vi "纳清浊度电极校准.vi"() -> ()   [LabVIEW 2016, in "斯坦道多参数.lvlib"]
uses:
  <vilib>/Utility/miscctls.llb/LVPointTypeDef.ctl
  <vilib>/Utility/miscctls.llb/LVPositionTypeDef.ctl
  <vilib>/Analysis/NI_AALBase.lvlib
panel:
  out "清扫间隔":u16
  out "清扫次数":u16
  in  "清扫模式":u16(ring) items=["自动清扫", "手动清扫", "启动一次清扫"]
  out "滤波设定":sgl
  out "第三点信号值":dbl
  out "第二点信号值":dbl
  out "第一点信号值":dbl
  in  "量程":u16(ring) items=["0-100", "0-500", "0-2000", "0-4000"]
  out "报警信息":string
  out "通讯状态":string
  out "第三点校准值":dbl
  out "标液3":sgl
  out "第二点校准值":dbl
  out "第一点校准值":dbl
  in  "校准停止":bool
  in  "校准启动":bool
  in  "校准模式":u16(ring)=1 items=["两点校准", "单点校准", "三点校准"]
  out "最小值":sgl format="%#.2f"
  out "最大值":sgl format="%#.2f"
  out "波形图表":dbl(graph) caption="历史曲线"
  out "mean":dbl caption="均值" format="%#.2f"
  out "standard deviation":dbl caption="标准差" format="%#.2f"
  out "变异系数":dbl format="%#.6f"
  out "测量值":sgl format="%#.2f"
  out "提示":string
  out "标液2":sgl
  out "标液1":sgl
  out "原始光强数值":u16 caption="信号值"
  out "温度":dbl format="%#.2f"
  # "浊度电极设定"
  # "℃"
  # "NTU"
  # "NTU"
  # "请选择校准模式:"
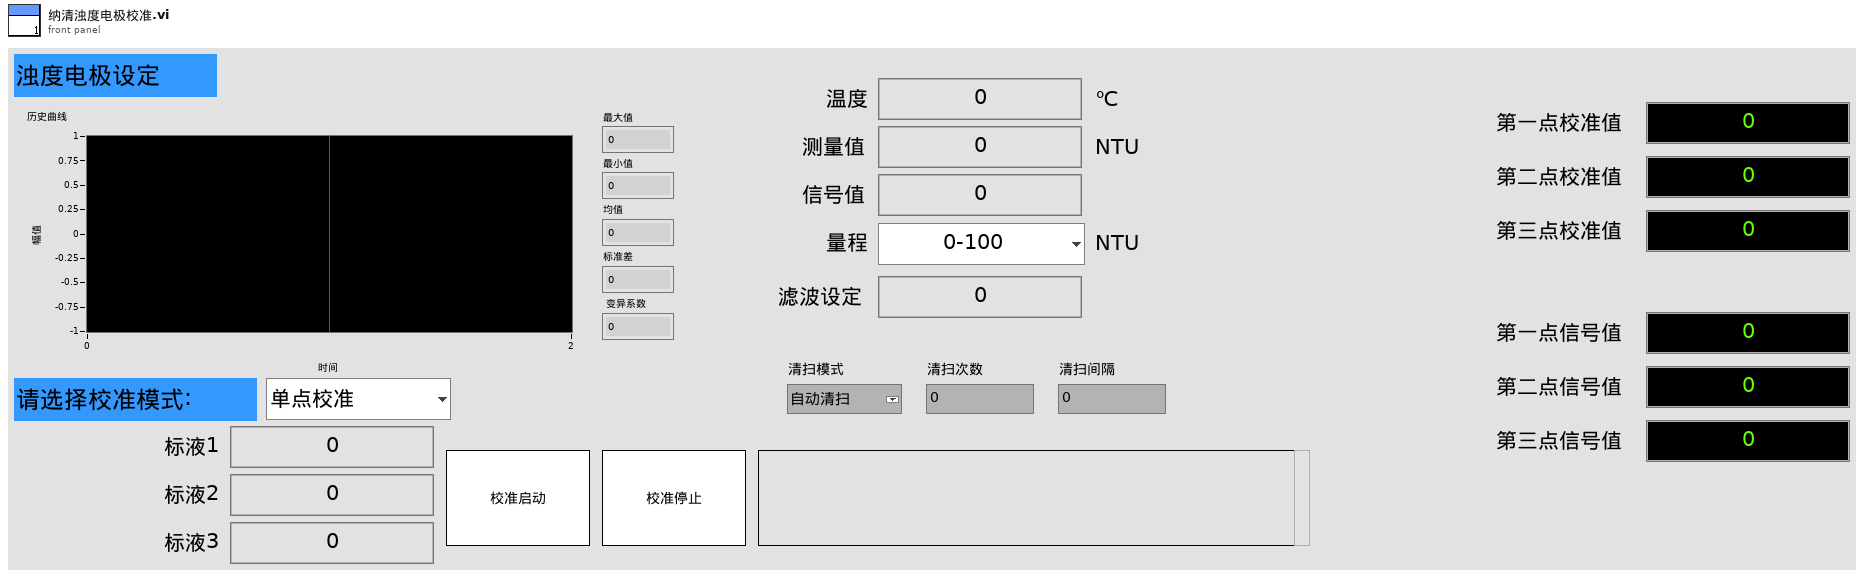
[diagram p1: front panel]
types:
  T1 = enum16{"pH", "DO", "Cond", "Turb", "ORP", "叶绿素a", "藻密度"}
  T2 = typedef "LVPointTypeDef.ctl" = cluster{"Horizontal":i16, "Vertical":i16}
  T3 = cluster{"报警码":u16, "浊度数值 NTU":sgl, "温度数据":sgl, "原始光强数值":u16, "量程":u16, "平均次数":u16, "清扫模式":u16, "清扫次数":u16, "清扫间隔分钟":u16, "0X000B_NC":string, "产品名称":string, "序列号":string, "硬件版本":string, "软件版本":string, "通讯地址":u16, "波特率":u16, "设备类型":u16, "0X0026_NC":string, "校准量程":u16, "第一点原始光强":u16, "第一点校准数据":sgl, "第二点原始光强":u16, "第二点校准数据":sgl, "第三点原始光强":u16, "第三点校准数据":sgl, "探头校准命令":u16, "温度校准参数":sgl, "温度校准命令":u16}
  T4 = cluster{"pH":u32, "DO":u32, "Cond":u32, "Turb":u32, "叶绿素a":u32, "藻密度":u32, "ORP":u32, "COD":u32}
  T5 = typedef "LVPositionTypeDef.ctl" = cluster{"Left":i32, "Top":i32}
  T6 = enum8{"Enabled", "Disabled", "Disabled and Grayed Out"}
  T7 = cluster{"ph":bool, "DO":bool, "Cond":bool, "Turb":bool, "叶绿素a":bool, "藻密度":bool, "ORP":bool, "COD":bool}
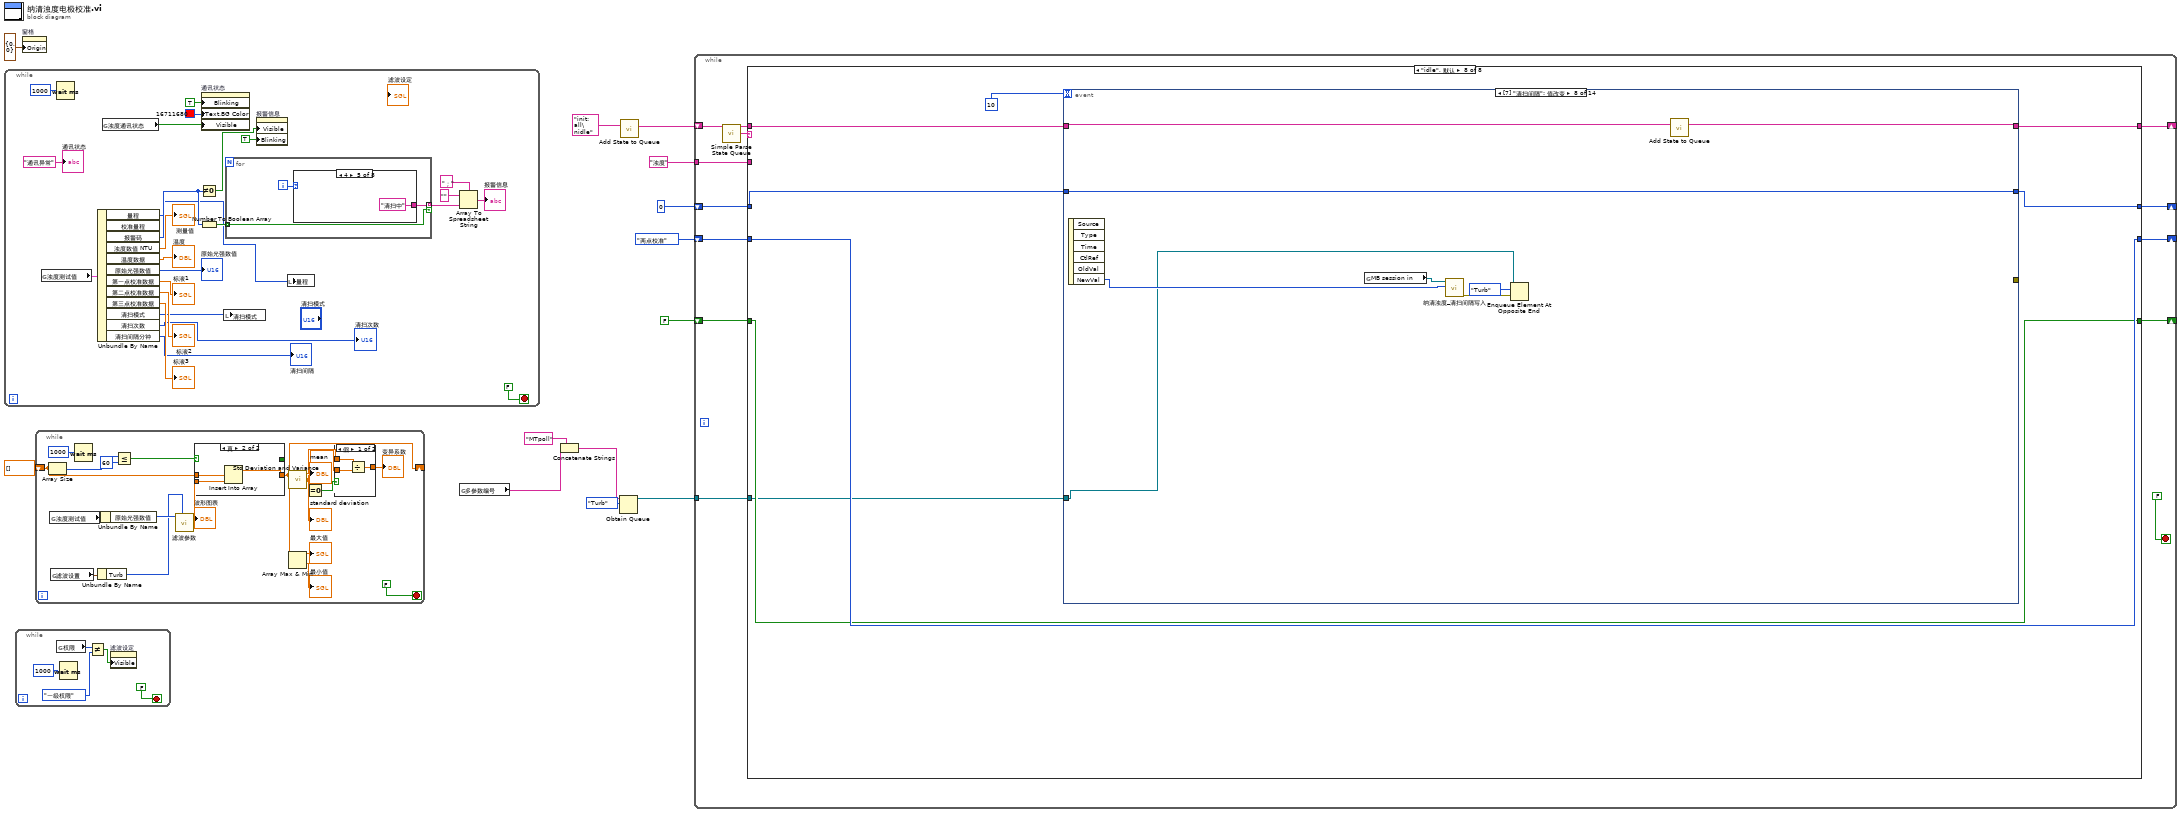
[diagram p0: block diagram]
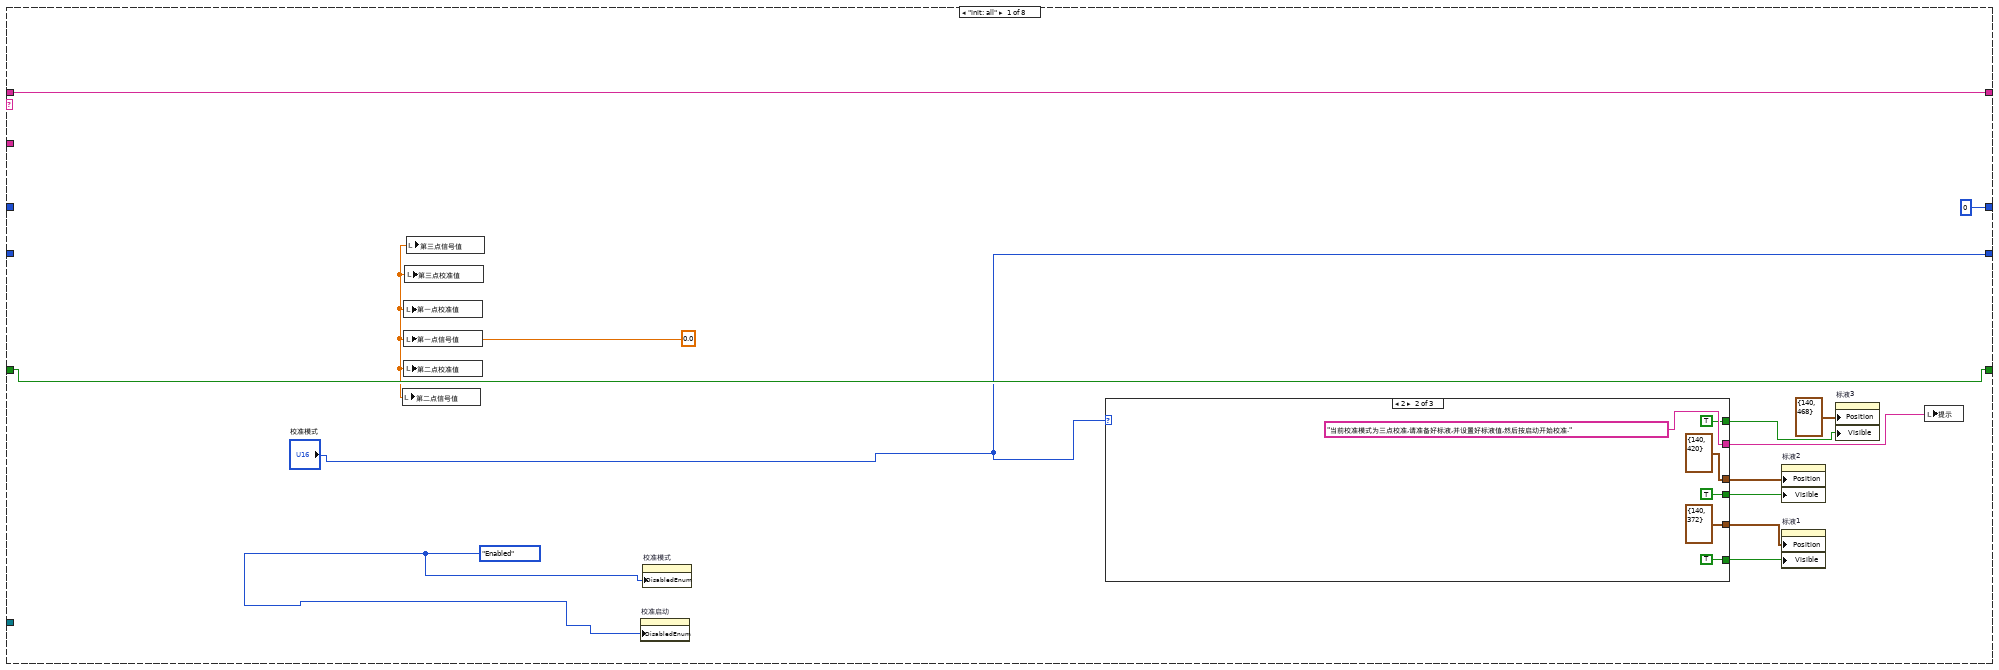
[diagram p2: hidden frame]
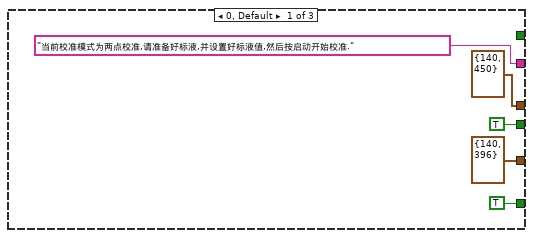
[diagram p3: hidden frame]
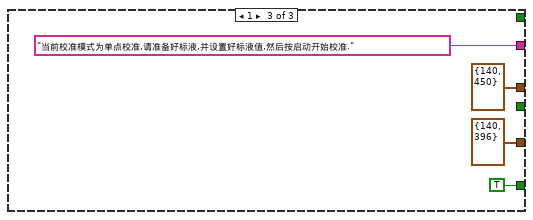
[diagram p4: hidden frame]
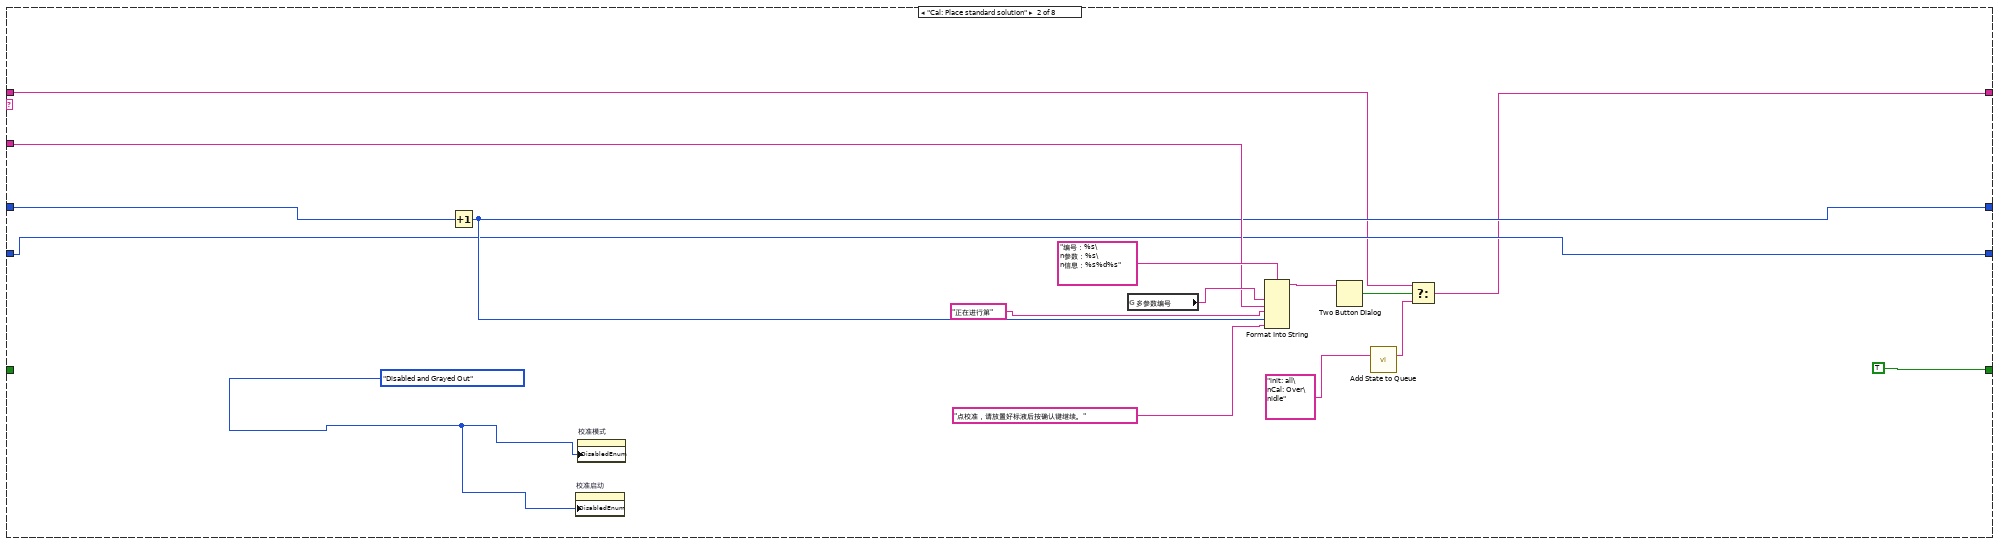
[diagram p5: hidden frame]
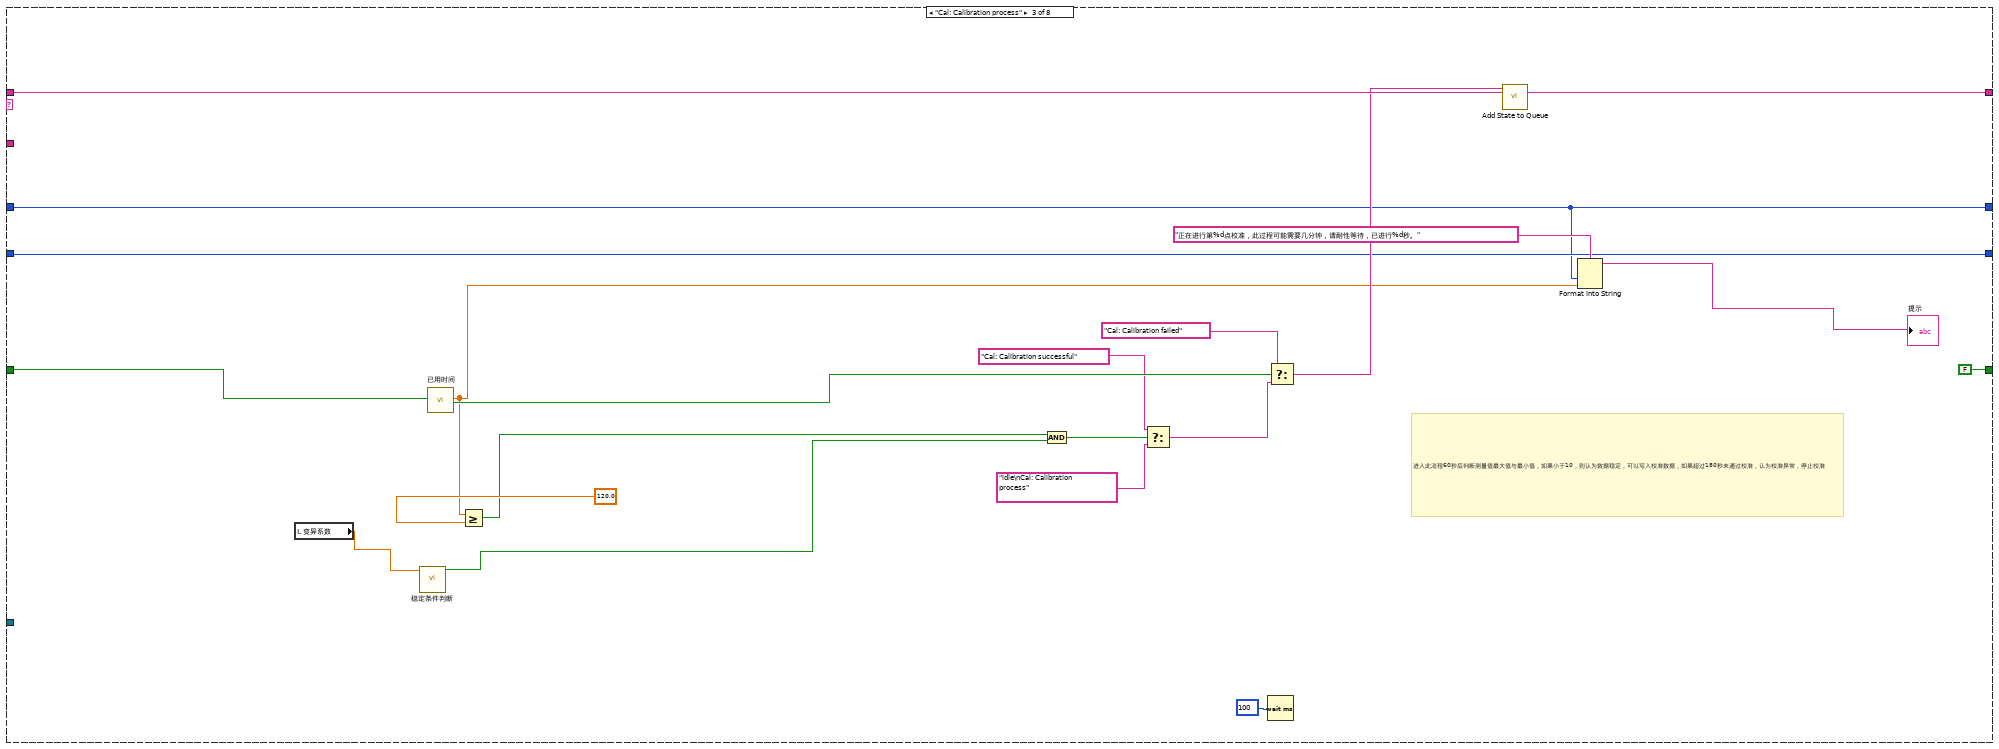
[diagram p6: hidden frame]
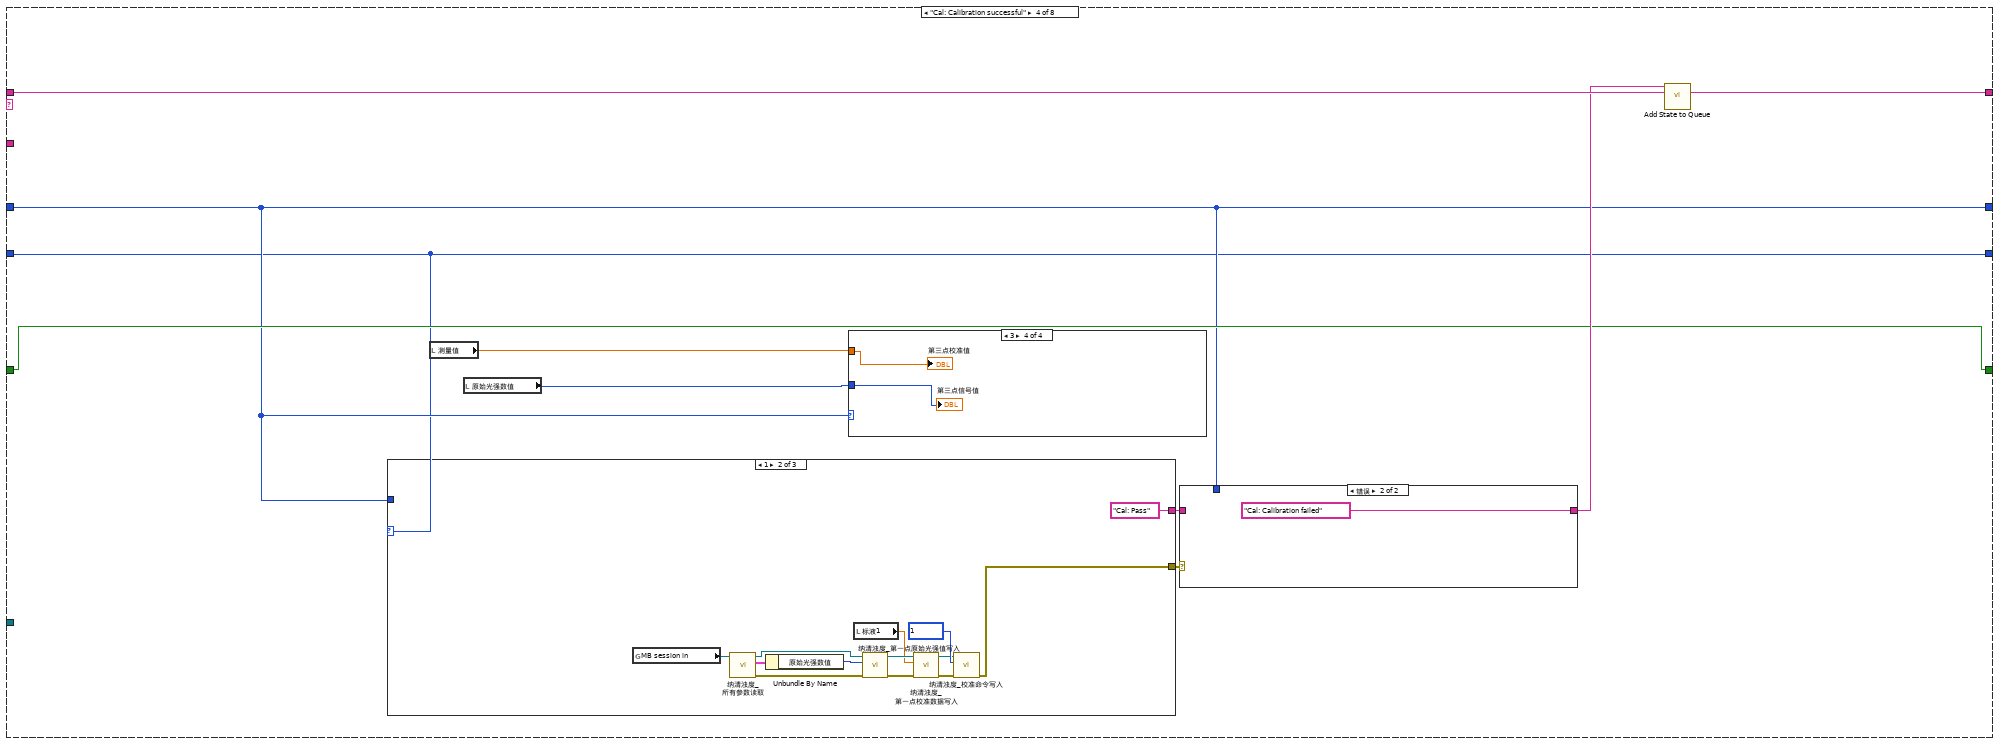
[diagram p7: hidden frame]
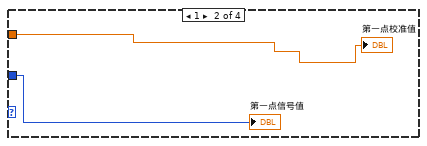
[diagram p9: hidden frame]
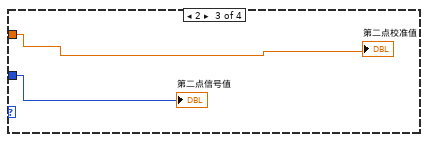
[diagram p10: hidden frame]
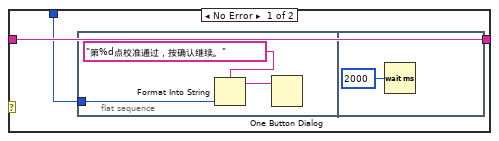
[diagram p11: hidden frame]
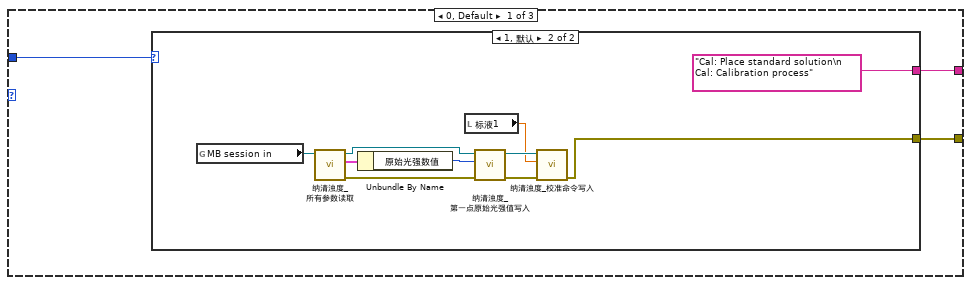
[diagram p12: hidden frame]
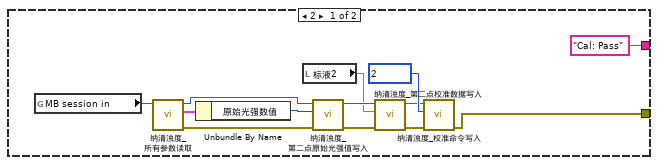
[diagram p13: hidden frame]
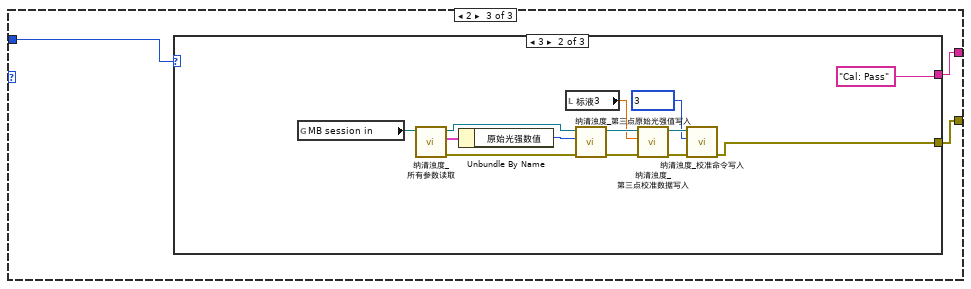
[diagram p14: hidden frame]
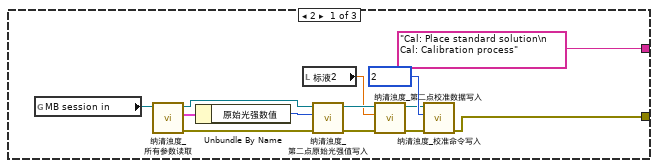
[diagram p15: hidden frame]
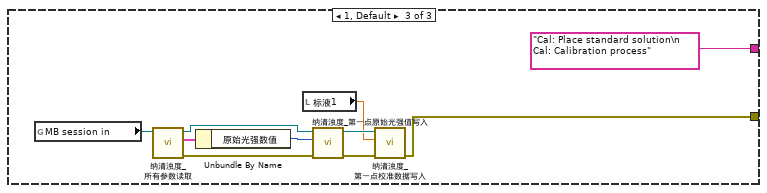
[diagram p16: hidden frame]
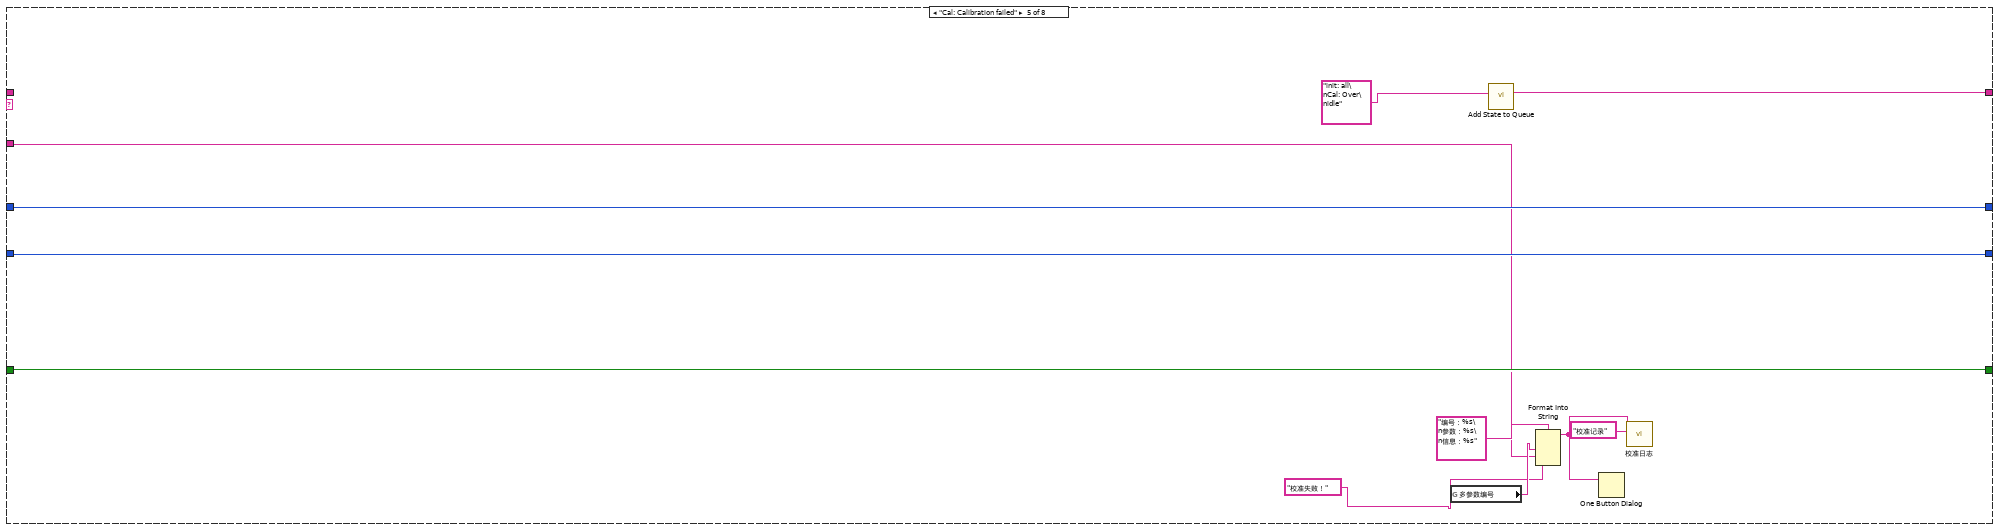
[diagram p17: hidden frame]
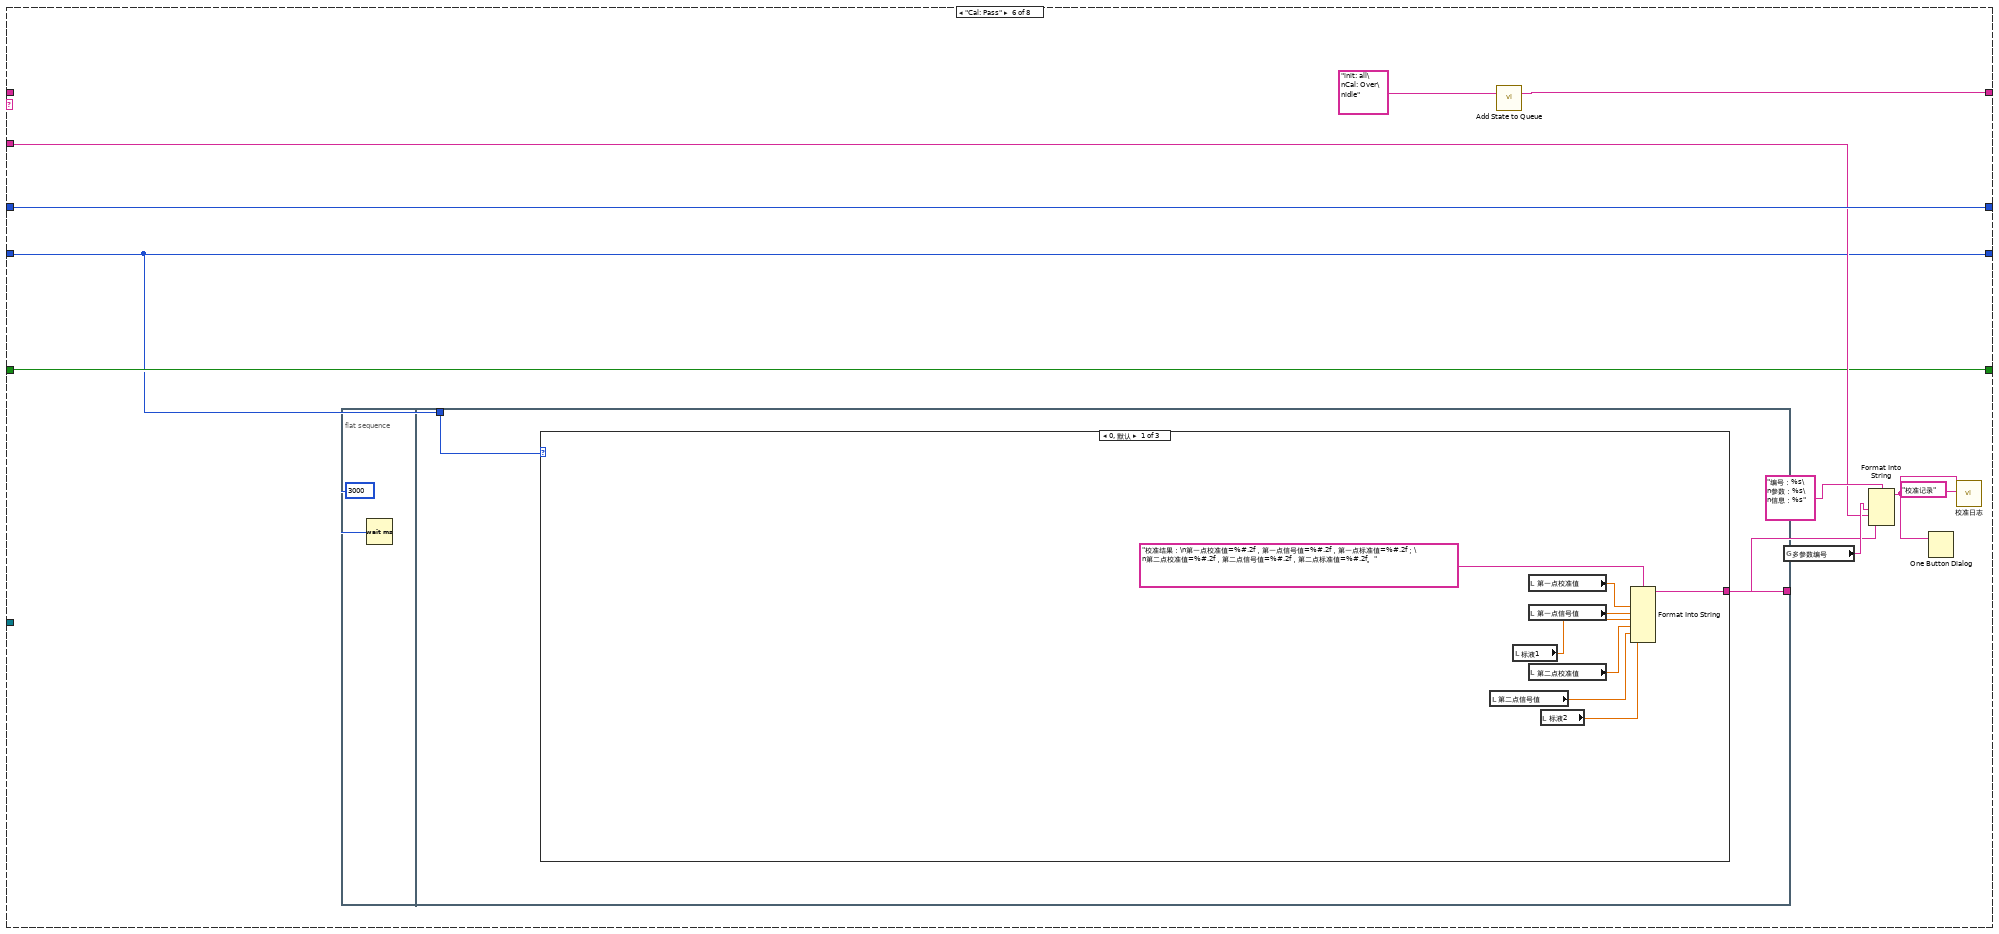
[diagram p18: hidden frame]
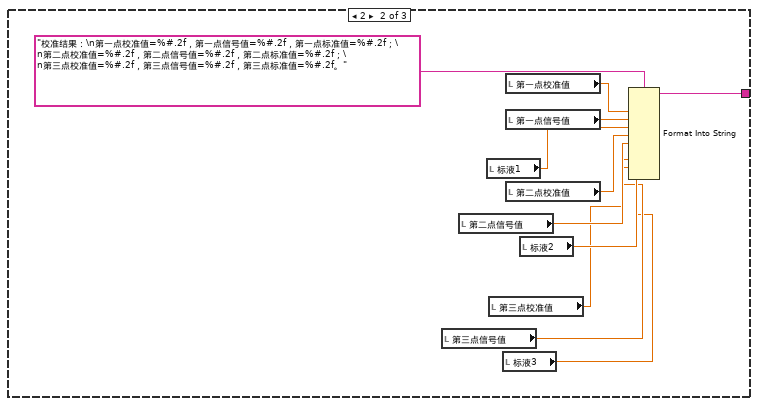
[diagram p19: hidden frame]
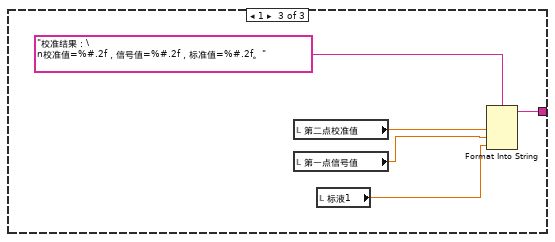
[diagram p20: hidden frame]
diagram:
  n1 = while {
    stop <- FALSE stop-if-true
    n2 = global read "纳清过程全局变量.vi" "浊度测试值"() -> (w36:T3)
    n3 = Wait (ms)(milliseconds to wait=u32 1000 ("等待时间（毫秒）")) -> ()  [unwired: 1 out]
    n4 = Unbundle By Name(w36) -> ("量程"=w17:u16, "报警码"=w18:u16, "浊度数值 NTU"=→"测量值":sgl, "温度数据"=→"温度":sgl, "原始光强数值"=→"原始光强数值":u16, "第一点校准数据"=→"标液1":sgl, "第二点校准数据"=→"标液2":sgl, "第三点校准数据"=→"标液3":sgl, "清扫模式"=w14:u16, "清扫次数"=→"清扫次数":u16, "清扫间隔分钟"=→"清扫间隔":u16)  [unwired: 1 out]
    n5 = global read "多参数全局变量.vi" "浊度通讯状态"() -> (w26:bool)
    n6 = Not Equal To 0?(x=w18) -> (x != 0?=w20:bool)
    n7 = Number To Boolean Array(number=w18) -> (Boolean array=w25:bool[])
    n8 = property on="通讯状态" class="Str"("Blinking"=TRUE ("闪烁"), "Text.BG Color"=u32 16711680, "Visible"=w26) -> ()  [unwired: 2 in, 2 out]
    n9 = local write "清扫模式"(w14) -> ()
    n10 = for {
      tunnel: w25 -> [w39] mode=indexing
      tunnel: [w40] -> w24 mode=indexing if=w39
      i -> [w41]
      n11 = case shown="4" w41 {
        tunnel: [_ "浊度超量程" "温度超量程" "光强信号超范围" "清扫中" "温度传感器故障" "电极故障" "内部电压基准故障"] -> w40
        frame Default {
        }
        frame 0 {
        }
        frame 2 {
        }
        frame 3 {
        }
        frame 4 {
        }
        frame 8 {
        }
        frame 9 {
        }
        frame 10 {
        }
      }
    }
    n12 = property on="报警信息" class="Str"("Visible"=w20, "Blinking"=TRUE ("闪烁")) -> ()  [unwired: 2 in, 2 out]
    n13 = local write "量程"(w17) -> ()
    n14 = Array To Spreadsheet String(delimiter (Tab)="；" ("分隔符(Tab)"), array=w24, 3:"" ("格式字符串")) -> (spreadsheet string=→"报警信息":string)
    "通讯状态" <- "通讯异常" ("当前串口")
  }
  n15 = while {
    stop <- FALSE stop-if-true
    n16 = global read "多参数全局变量.vi" "权限"() -> (w52:enum16{"一级权限", "二级权限", "三级权限"})
    n17 = Wait (ms)(milliseconds to wait=u32 1000 ("等待时间（毫秒）")) -> ()  [unwired: 1 out]
    n18 = Not Equal?(x=w52, y=enum16{"一级权限", "二级权限", "三级权限"}."一级权限") -> (x != y?=w49:bool)
    n19 = property on="滤波设定" class="DigNum (严格)"("Visible"=w49) -> ()  [unwired: 2 in, 2 out]
  }
  n20 = property on="窗格" class="Pane"("Origin"=T2 {"Horizontal"=0, "Vertical"=0} ("原点")) -> ()  [unwired: 2 in, 2 out]
  n21 = while {
    shift-right: [w61] -> _
    shift-left: sgl[] [] -> [w67]
    stop <- FALSE stop-if-true
    n22 = Array Size(array=w67) -> (size(s)=w69:i32)
    n23 = global read "纳清过程全局变量.vi" "浊度测试值"() -> (w58:T3)
    n24 = global read "断电保存变量.vi" "滤波设置"() -> (w55:T4)
    n25 = Wait (ms)(milliseconds to wait=u32 1000 ("等待时间（毫秒）")) -> ()  [unwired: 1 out]
    n26 = Unbundle By Name(w55) -> ("Turb"=w54:u32)
    n27 = Unbundle By Name(w58) -> ("原始光强数值"=w57:u16)
    n28 = Less Or Equal?(x=w69, y=60) -> (x <= y?=w68:bool)
    n29 = call "滤波参数.vi"("滤波次数"=w54, "x"=w57) -> ("mode"=w56:dbl)  [unwired: 9 in]
    "波形图表" <- w56
    n30 = case shown="真" w68 {
      tunnel: w67 -> [w80 w83]
      tunnel: w56 -> [w78 w82]
      tunnel: [w76 w81] -> w61
      tunnel: [TRUE _] -> _
      frame False {
        n31 = Replace Array Subset(array=w80, new element=w78) -> (w79:sgl[])  [unwired: 1 in]
        n32 = Rotate 1D Array(1:w79, 2:-1 ("n")) -> (0:w76:sgl[])
      }
      frame True {
        n33 = Insert Into Array(array=w83, new element=w82) -> (w81:sgl[])  [unwired: 1 in]
      }
    }
    n34 = call <vilib>:"Std Deviation and Variance.vi"("X"=w61) -> ("mean"=w65:dbl, "standard deviation"=w64:dbl)  [unwired: 1 in, 1 out]
    "mean" <- w65
    "standard deviation" <- w64
    n35 = Array Max & Min(array=w61) -> (max value=→"最大值":sgl, min value=→"最小值":sgl)  [unwired: 2 out]
    n36 = Equal To 0?(x=w65) -> (x = 0?=w66:bool)
    n37 = case shown="假" w66 {
      tunnel: w64 -> [w74 _]
      tunnel: [w73 _] -> w63
      tunnel: w65 -> [w72 _]
      frame False {
        n38 = Divide(x=w74, y=w72) -> (x/y=w73:dbl)
      }
      frame True {
      }
    }
    "变异系数" <- w63
  }
  n39 = global read "多参数全局变量.vi" "多参数编号"() -> (w2:string)
  n40 = Concatenate Strings("MTpoll" ("名称（未命名）"), w2) -> (w4:string)
  n41 = Obtain Queue(name (unnamed)=w4, element data type=T1."Turb" ("枚举")) -> (queue out=w1:refnum<queue>)  [unwired: 3 in, 2 out]
  n42 = call "Add State to Queue.vi"("State(s) In (\"\")"="init: all\nidle" ("State(s) In (\"\")")) -> ("States Out"=w10:string)  [unwired: 14 in]
  n43 = while {
    shift-right: [w92] -> _
    shift-left: w10 -> [w96]
    shift-right: [w89] -> _
    shift-left: 0 -> [w91]
    tunnel: "浊度" ("State(s) In (\"\")") -> [w90]
    shift-right: [w87] -> _
    shift-left: enum16{"两点校准", "单点校准", "三点校准"}."两点校准" ("校准模式") -> [w88]
    shift-right: [w85] -> _
    shift-left: FALSE -> [w86]
    tunnel: w1 -> [w84]
    stop <- FALSE stop-if-true
    n44 = call "Simple Parse State Queue.vi"("State Queue"=w96) -> ("Remain States"=w93:string, "Next State"=w94:string)  [unwired: 13 in]
    n45 = case shown="\"idle\", 默认" w94 {
      tunnel: w93 -> [w109 w128 w160 w169 _ _ w318 w326]
      tunnel: [w109 w127 w159 w168 w270 w275 w318 w325] -> w92
      tunnel: w91 -> [_ w136 w145 w163 w273 w284 w317 w323]
      tunnel: w90 -> [_ w137 _ _ w264 w280 _ _]
      tunnel: [0 w134 w145 w163 w273 w284 w317 w324] -> w89
      tunnel: w88 -> [_ w133 w146 w162 w272 w276 w316 w322]
      tunnel: ["校准模式" w133 w146 w162 w272 w276 w316 w322] -> w87
      tunnel: w86 -> [w107 _ w148 w164 w271 w279 w315 w320]
      tunnel: [w107 TRUE FALSE w164 w271 w279 w315 w320] -> w85
      tunnel: w84 -> [_ _ _ _ _ _ _ w319]
      frame "init: all" {
        w105 = T6."Enabled" ("禁用")
        w106 = 0.0 ("第一点校准值")
        n46 = local write "第二点信号值"(w106) -> ()
        n47 = local write "第一点校准值"(w106) -> ()
        n48 = local write "第一点信号值"(w106) -> ()
        n49 = local write "第二点校准值"(w106) -> ()
        n50 = local write "第三点校准值"(w106) -> ()
        n51 = local write "第三点信号值"(w106) -> ()
        n52 = property on="校准启动" class="Bool"("DisabledEnum"=w105) -> ()  [unwired: 2 in, 2 out]
        n53 = property on="校准模式" class="Ring (严格)"("DisabledEnum"=w105) -> ()  [unwired: 2 in, 2 out]
        n54 = case shown="2" "校准模式" {
          tunnel: ["当前校准模式为两点校准,请准备好标液,并设置好标液值,然后按启动开始校准." ("提示") "当前校准模式为三点校准,请准备好标液,并设置好标液值,然后按启动开始校准." ("提示") "当前校准模式为单点校准,请准备好标液,并设置好标液值,然后按启动开始校准." ("提示")] -> w97
          tunnel: [TRUE ("可见") TRUE ("可见") _] -> w102
          tunnel: [T5 {"Left"=140, "Top"=396} ("位置") T5 {"Left"=140, "Top"=372} ("位置") T5 {"Left"=140, "Top"=396} ("位置")] -> w99
          tunnel: [T5 {"Left"=140, "Top"=450} ("位置 2") T5 {"Left"=140, "Top"=420} ("位置 2") T5 {"Left"=140, "Top"=450} ("位置 2")] -> w100
          tunnel: [_ TRUE ("可见") _] -> w103
          tunnel: [TRUE ("可见") TRUE ("可见") TRUE ("可见")] -> w104
          frame 0, Default {
          }
          frame 2 {
          }
          frame 1 {
          }
        }
        n55 = property on="标液2" class="DigNum (严格)"("Position"=w100, "Visible"=w102) -> ()  [unwired: 2 in, 2 out]
        n56 = property on="标液1" class="DigNum (严格)"("Position"=w99, "Visible"=w104) -> ()  [unwired: 2 in, 2 out]
        n57 = property on="标液3" class="DigNum (严格)"("Position"=T5 {"Left"=140, "Top"=468} ("位置 3"), "Visible"=w103) -> ()  [unwired: 2 in, 2 out]
        n58 = local write "提示"(w97) -> ()
      }
      frame "Cal: Place standard solution" {
        w126 = T6."Disabled and Grayed Out" ("禁用")
        n59 = Increment(x=w136) -> (x+1=w134:i32)
        n60 = property on="校准启动" class="Bool"("DisabledEnum"=w126) -> ()  [unwired: 2 in, 2 out]
        n61 = property on="校准模式" class="Ring (严格)"("DisabledEnum"=w126) -> ()  [unwired: 2 in, 2 out]
        n62 = global read "多参数全局变量.vi" "多参数编号"() -> (w139:string)
        n63 = Format Into String(format string="编号：%s\n参数：%s\n信息：%s%d%s" ("格式字符串"), w139, w137, "正在进行第" ("消息"), w134, "点校准，请放置好标液后按确认键继续。" ("消息")) -> (resulting string=w131:string)  [unwired: 2 in, 1 out]
        n64 = Two Button Dialog(message=w131) -> (T button?=w130:bool)  [unwired: 2 in]
        n65 = call "Add State to Queue.vi"("State(s) In (\"\")"="init: all\nCal: Over\nidle" ("State(s) In (\"\")")) -> ("States Out"=w129:string)  [unwired: 14 in]
        n66 = Select(t=w128, s=w130, f=w129) -> (s? t:f=w127:string)
      }
      frame "Cal: Calibration process" {
        # "进入此流程60秒后判断测量值最大值与最小值，如果小于10，则认为数据稳定，可以写入校准数据，如果超过180秒未通过校准，认为校准异常，停止校准"
        n67 = local read "变异系数"() -> (w142:dbl)
        n68 = call "稳定条件判断.vi"("变异系数"=w142) -> ("布尔"=w141:bool)  [unwired: 10 in]
        n69 = call "已用时间"("Reset"=w148) -> ("Elapsed Time (s)"=w144:dbl, "Time has Elapsed"=w161:bool)  [unwired: 11 in, 6 out]
        n70 = Greater Or Equal?(x=w144, y=120.0) -> (x >= y?=w156:bool)
        n71 = And(x=w156, y=w141) -> (x .and. y?=w153:bool)
        n72 = Select(t="Cal: Calibration successful" ("State(s) In (\"\")"), s=w153, f="idle\nCal: Calibration process" ("State(s) In (\"\")")) -> (s? t:f=w152:string)
        n73 = Wait (ms)(milliseconds to wait=u32 100 ("等待时间（毫秒）")) -> ()  [unwired: 1 out]
        n74 = Select(t="Cal: Calibration failed" ("State(s) In (\"\")"), s=w161, f=w152) -> (s? t:f=w151:string)
        n75 = call "Add State to Queue.vi"("State(s) In Front (\"\")"=w151, "State(s) In (\"\")"=w160) -> ("States Out"=w159:string)  [unwired: 13 in]
        n76 = Format Into String(format string="正在进行第%d点校准，此过程可能需要几分钟，请耐性等待，已进行%d秒。" ("格式字符串"), w145, w144) -> (resulting string=→"提示":string)  [unwired: 2 in, 1 out]
      }
      frame "Cal: Calibration successful" {
        n77 = case shown="1" w162 {
          tunnel: [w187 w211 w224] -> w171
          tunnel: [w186 "Cal: Pass" ("State(s) In (\"\")") w225] -> w170
          tunnel: w163 -> [w185 _ w226]
          frame 0, Default {
            n78 = case shown="1, 默认" w185 {
              tunnel: [w188 w201] -> w187
              tunnel: ["Cal: Pass" ("State(s) In (\"\")") "Cal: Place standard solution\n Cal: Calibration process" ("State(s) In (\"\")")] -> w186
              frame 2 {
                n79 = global read "多参数全局变量.vi" "MB session in"() -> (w196:refnum<class "MB_Master.lvclass">)
                n80 = call "纳清浊度_所有参数读取.vi"("MB session in"=w196) -> ("error out"=w198:errorcluster, "输出值"=w195:T3, "MB session out"=w197:refnum<class "MB_Master.lvclass">)  [unwired: 8 in]
                n81 = Unbundle By Name(w195) -> ("原始光强数值"=w194:u16)
                n82 = local read "标液2"() -> (w189:sgl)
                n83 = call "纳清浊度_第二点原始光强值写入.vi"("error in (no error)"=w198, "数值"=w194, "MB session in"=w197) -> ("error out"=w193:errorcluster, "MB session out"=w192:refnum<class "MB_Master.lvclass">)  [unwired: 7 in]
                n84 = call "纳清浊度_第二点校准数据写入.vi"("error in (no error)"=w193, "数值"=w189, "MB session in"=w192) -> ("error out"=w191:errorcluster, "MB session out"=w190:refnum<class "MB_Master.lvclass">)  [unwired: 7 in]
                n85 = call "纳清浊度_校准命令写入.vi"("error in (no error)"=w191, "数值"=u16 2 ("starting address"), "MB session in"=w190) -> ("error out"=w188:errorcluster)  [unwired: 7 in, 1 out]
              }
              frame 1, Default {
                n86 = global read "多参数全局变量.vi" "MB session in"() -> (w207:refnum<class "MB_Master.lvclass">)
                n87 = call "纳清浊度_所有参数读取.vi"("MB session in"=w207) -> ("error out"=w209:errorcluster, "输出值"=w206:T3, "MB session out"=w208:refnum<class "MB_Master.lvclass">)  [unwired: 8 in]
                n88 = Unbundle By Name(w206) -> ("原始光强数值"=w205:u16)
                n89 = local read "标液1"() -> (w202:sgl)
                n90 = call "纳清浊度_第一点原始光强值写入.vi"("error in (no error)"=w209, "数值"=w205, "MB session in"=w208) -> ("error out"=w204:errorcluster, "MB session out"=w203:refnum<class "MB_Master.lvclass">)  [unwired: 7 in]
                n91 = call "纳清浊度_校准命令写入.vi"("error in (no error)"=w204, "数值"=w202, "MB session in"=w203) -> ("error out"=w201:errorcluster)  [unwired: 7 in, 1 out]
              }
            }
          }
          frame 1 {
            n92 = global read "多参数全局变量.vi" "MB session in"() -> (w219:refnum<class "MB_Master.lvclass">)
            n93 = call "纳清浊度_所有参数读取.vi"("MB session in"=w219) -> ("error out"=w221:errorcluster, "输出值"=w218:T3, "MB session out"=w220:refnum<class "MB_Master.lvclass">)  [unwired: 8 in]
            n94 = Unbundle By Name(w218) -> ("原始光强数值"=w217:u16)
            n95 = local read "标液1"() -> (w212:sgl)
            n96 = call "纳清浊度_第一点原始光强值写入.vi"("error in (no error)"=w221, "数值"=w217, "MB session in"=w220) -> ("error out"=w216:errorcluster, "MB session out"=w215:refnum<class "MB_Master.lvclass">)  [unwired: 7 in]
            n97 = call "纳清浊度_第一点校准数据写入.vi"("error in (no error)"=w216, "数值"=w212, "MB session in"=w215) -> ("error out"=w214:errorcluster, "MB session out"=w213:refnum<class "MB_Master.lvclass">)  [unwired: 7 in]
            n98 = call "纳清浊度_校准命令写入.vi"("error in (no error)"=w214, "数值"=u16 1 ("starting address"), "MB session in"=w213) -> ("error out"=w211:errorcluster)  [unwired: 7 in, 1 out]
          }
          frame 2 {
            n99 = case shown="3" w226 {
              tunnel: [w228 w240 w253] -> w224
              tunnel: ["Cal: Place standard solution\n Cal: Calibration process" ("State(s) In (\"\")") "Cal: Pass" ("State(s) In (\"\")") "Cal: Place standard solution\n Cal: Calibration process" ("State(s) In (\"\")")] -> w225
              frame 2 {
                n100 = global read "多参数全局变量.vi" "MB session in"() -> (w236:refnum<class "MB_Master.lvclass">)
                n101 = call "纳清浊度_所有参数读取.vi"("MB session in"=w236) -> ("error out"=w238:errorcluster, "输出值"=w235:T3, "MB session out"=w237:refnum<class "MB_Master.lvclass">)  [unwired: 8 in]
                n102 = Unbundle By Name(w235) -> ("原始光强数值"=w234:u16)
                n103 = local read "标液2"() -> (w229:sgl)
                n104 = call "纳清浊度_第二点原始光强值写入.vi"("error in (no error)"=w238, "数值"=w234, "MB session in"=w237) -> ("error out"=w233:errorcluster, "MB session out"=w232:refnum<class "MB_Master.lvclass">)  [unwired: 7 in]
                n105 = call "纳清浊度_第二点校准数据写入.vi"("error in (no error)"=w233, "数值"=w229, "MB session in"=w232) -> ("error out"=w231:errorcluster, "MB session out"=w230:refnum<class "MB_Master.lvclass">)  [unwired: 7 in]
                n106 = call "纳清浊度_校准命令写入.vi"("error in (no error)"=w231, "数值"=u16 2 ("starting address"), "MB session in"=w230) -> ("error out"=w228:errorcluster)  [unwired: 7 in, 1 out]
              }
              frame 3 {
                n107 = global read "多参数全局变量.vi" "MB session in"() -> (w249:refnum<class "MB_Master.lvclass">)
                n108 = call "纳清浊度_所有参数读取.vi"("MB session in"=w249) -> ("error out"=w251:errorcluster, "输出值"=w248:T3, "MB session out"=w250:refnum<class "MB_Master.lvclass">)  [unwired: 8 in]
                n109 = Unbundle By Name(w248) -> ("原始光强数值"=w247:u16)
                n110 = local read "标液3"() -> (w241:sgl)
                n111 = call "纳清浊度_第三点原始光强值写入.vi"("error in (no error)"=w251, "数值"=w247, "MB session in"=w250) -> ("error out"=w246:errorcluster, "MB session out"=w245:refnum<class "MB_Master.lvclass">)  [unwired: 7 in]
                n112 = call "纳清浊度_第三点校准数据写入.vi"("error in (no error)"=w246, "数值"=w241, "MB session in"=w245) -> ("error out"=w244:errorcluster, "MB session out"=w243:refnum<class "MB_Master.lvclass">)  [unwired: 7 in]
                n113 = call "纳清浊度_校准命令写入.vi"("error in (no error)"=w244, "数值"=u16 3 ("starting address"), "MB session in"=w243) -> ("error out"=w240:errorcluster)  [unwired: 7 in, 1 out]
              }
              frame 1, Default {
                n114 = global read "多参数全局变量.vi" "MB session in"() -> (w259:refnum<class "MB_Master.lvclass">)
                n115 = call "纳清浊度_所有参数读取.vi"("MB session in"=w259) -> ("error out"=w261:errorcluster, "输出值"=w258:T3, "MB session out"=w260:refnum<class "MB_Master.lvclass">)  [unwired: 8 in]
                n116 = Unbundle By Name(w258) -> ("原始光强数值"=w257:u16)
                n117 = local read "标液1"() -> (w254:sgl)
                n118 = call "纳清浊度_第一点原始光强值写入.vi"("error in (no error)"=w261, "数值"=w257, "MB session in"=w260) -> ("error out"=w256:errorcluster, "MB session out"=w255:refnum<class "MB_Master.lvclass">)  [unwired: 7 in]
                n119 = call "纳清浊度_第一点校准数据写入.vi"("error in (no error)"=w256, "数值"=w254, "MB session in"=w255) -> ("error out"=w253:errorcluster)  [unwired: 7 in, 1 out]
              }
            }
          }
        }
        n120 = local read "测量值"() -> (w165:sgl)
        n121 = local read "原始光强数值"() -> (w166:u16)
        n122 = case shown="3" w163 {
          tunnel: w166 -> [_ w173 w175 w176]
          tunnel: w165 -> [_ w172 w174 w177]
          frame 0, Default {
          }
          frame 1 {
            "第一点信号值" <- w173
            "第一点校准值" <- w172
          }
          frame 2 {
            "第二点信号值" <- w175
            "第二点校准值" <- w174
          }
          frame 3 {
            "第三点校准值" <- w177
            "第三点信号值" <- w176
          }
        }
        n123 = case shown="错误" w171 {
          tunnel: w170 -> [w179 _]
          tunnel: [w179 "Cal: Calibration failed" ("State(s) In (\"\")")] -> w167
          tunnel: w163 -> [w178 _]
          frame No Error {
            n124 = flat-sequence {
              tunnel: w178 -> [w180]
              frame #0 {
                n125 = Format Into String(format string="第%d点校准通过，按确认继续。" ("格式字符串"), w180) -> (resulting string=w182:string)  [unwired: 2 in, 1 out]
                n126 = One Button Dialog(message=w182) -> ()  [unwired: 1 in, 1 out]
              }
              frame #1 {
                n127 = Wait (ms)(milliseconds to wait=u32 2000 ("等待时间（毫秒）")) -> ()  [unwired: 1 out]
              }
            }
          }
          frame Error {
          }
        }
        n128 = call "Add State to Queue.vi"("State(s) In Front (\"\")"=w167, "State(s) In (\"\")"=w169) -> ("States Out"=w168:string)  [unwired: 13 in]
      }
      frame "Cal: Calibration failed" {
        n129 = global read "多参数全局变量.vi" "多参数编号"() -> (w267:string)
        n130 = call "Add State to Queue.vi"("State(s) In (\"\")"="init: all\nCal: Over\nidle" ("State(s) In (\"\")")) -> ("States Out"=w270:string)  [unwired: 14 in]
        n131 = Format Into String(format string="编号：%s\n参数：%s\n信息：%s" ("格式字符串"), w267, w264, "校准失败！" ("消息")) -> (resulting string=w266:string)  [unwired: 2 in, 1 out]
        n132 = One Button Dialog(message=w266) -> ()  [unwired: 1 in, 1 out]
        n133 = call "校准日志.vi"("table"="校准记录", "日志信息"=w266) -> ()  [unwired: 9 in, 1 out]
      }
      frame "Cal: Pass" {
        n134 = flat-sequence {
          tunnel: [w287] -> w277
          tunnel: w276 -> [w286]
          frame #0 {
            n135 = Wait (ms)(milliseconds to wait=u32 3000 ("等待时间（毫秒）")) -> ()  [unwired: 1 out]
          }
          frame #1 {
            n136 = case shown="0, 默认" w286 {
              tunnel: [w295 w306 w311] -> w287
              frame 0, Default {
                n137 = local read "第二点信号值"() -> (w289:dbl)
                n138 = local read "标液1"() -> (w291:sgl)
                n139 = local read "第一点校准值"() -> (w293:dbl)
                n140 = local read "第一点信号值"() -> (w294:dbl)
                n141 = local read "第二点校准值"() -> (w290:dbl)
                n142 = local read "标液2"() -> (w288:sgl)
                n143 = Format Into String(format string="校准结果：\n第一点校准值=%#.2f，第一点信号值=%#.2f，第一点标准值=%#.2f；\n第二点校准值=%#.2f，第二点信号值=%#.2f，第二点标准值=%#.2f。" ("提示"), w293, w294, w291, w290, w289, w288) -> (resulting string=w295:string)  [unwired: 2 in, 1 out]
              }
              frame 2 {
                n144 = local read "第三点信号值"() -> (w297:dbl)
                n145 = local read "第二点信号值"() -> (w300:dbl)
                n146 = local read "标液1"() -> (w302:sgl)
                n147 = local read "第三点校准值"() -> (w298:dbl)
                n148 = local read "标液3"() -> (w296:sgl)
                n149 = local read "第一点校准值"() -> (w304:dbl)
                n150 = local read "第一点信号值"() -> (w305:dbl)
                n151 = local read "第二点校准值"() -> (w301:dbl)
                n152 = local read "标液2"() -> (w299:sgl)
                n153 = Format Into String(format string="校准结果：\n第一点校准值=%#.2f，第一点信号值=%#.2f，第一点标准值=%#.2f；\n第二点校准值=%#.2f，第二点信号值=%#.2f，第二点标准值=%#.2f；\n第三点校准值=%#.2f，第三点信号值=%#.2f，第三点标准值=%#.2f。" ("提示"), w304, w305, w302, w301, w300, w299, w298, w297, w296) -> (resulting string=w306:string)  [unwired: 2 in, 1 out]
              }
              frame 1 {
                n154 = local read "第二点校准值"() -> (w310:dbl)
                n155 = local read "第一点信号值"() -> (w308:dbl)
                n156 = local read "标液1"() -> (w307:sgl)
                n157 = Format Into String(format string="校准结果：\n校准值=%#.2f，信号值=%#.2f，标准值=%#.2f。" ("提示"), w310, w308, w307) -> (resulting string=w311:string)  [unwired: 2 in, 1 out]
              }
            }
          }
        }
        n158 = call "Add State to Queue.vi"("State(s) In (\"\")"="init: all\nCal: Over\nidle" ("State(s) In (\"\")")) -> ("States Out"=w275:string)  [unwired: 14 in]
        n159 = global read "多参数全局变量.vi" "多参数编号"() -> (w281:string)
        n160 = Format Into String(format string="编号：%s\n参数：%s\n信息：%s" ("格式字符串"), w281, w280, w277) -> (resulting string=w278:string)  [unwired: 2 in, 1 out]
        n161 = One Button Dialog(message=w278) -> ()  [unwired: 1 in, 1 out]
        n162 = call "校准日志.vi"("table"="校准记录", "日志信息"=w278) -> ()  [unwired: 9 in, 1 out]
      }
      frame "Cal: Over" {
        n163 = global read "多参数全局变量.vi" "校准运行状态"() -> (w313:T7)
        n164 = Bundle By Name(cluster=w313, "Turb"=FALSE ("Cond")) -> (w314:T7)
        n165 = global write "多参数全局变量.vi" "校准运行状态"(w314) -> ()
      }
      frame "idle", Default {
        n166 = event shown="[7] \"清扫间隔\": 值改变" {
          selector: _ -> [_ _ _ _ _ _ _ _ _ _ _ _ _ _]
          dyn-events: _ -> [_ _ _ _ _ _ _ _ _ _ _ _ _ _]
          timeout: 10 -> [_ _ _ _ _ _ _ _ _ _ _ _ _ _]
          tunnel: w326 -> [w329 w333 w338 w345 w351 w359 w367 w375 w383 w391 w396 w405 w420 _]
          tunnel: [w328 w332 w339 w346 w355 w363 w371 w379 w387 w395 w398 w409 w419 w422] -> w325
          tunnel: [w327 w330 w340 w347 w354 w362 w370 w378 w386 w394 w397 w408 w417 w423] -> w324
          tunnel: w323 -> [w327 w330 w340 w347 w354 w362 w370 w378 w386 w394 w397 w408 w417 w423]
          tunnel: [_ _ _ _ _ _ _ _ _ _ _ _ w410 _] -> _
          tunnel: w319 -> [_ _ _ _ w349 w357 w365 w373 w381 w389 _ w403 _ _]
          event Timeout {
            n167 = event-data() -> ()  [unwired: 1 in, 3 out]
            n168 = call "Add State to Queue.vi"("State(s) In (\"\")"=w329) -> ("States Out"=w328:string)  [unwired: 14 in]
          }
          event "校准模式": Value Change {
            n169 = event-data() -> ()  [unwired: 1 in, 6 out]
            n170 = call "Add State to Queue.vi"("State(s) In (\"\")"=w333, "State(s) At Back (\"\")"="init: all\nidle" ("State(s) In (\"\")")) -> ("States Out"=w332:string)  [unwired: 13 in]
          }
          event "标液1", "标液2", "标液3", "滤波设定": Mouse Down {
            n171 = event-data() -> ("CtlRef"=w337:refnum<vi>)  [unwired: 1 in, 7 out]
            n172 = property class="DigNum (严格)"(reference=w337) -> (reference out=w334:refnum<vi>, "Value"=w335:sgl)  [unwired: 1 in, 1 out]
            n173 = call "数字键盘.vi"("OldNumber"=w335) -> ("NewNumber"=w336:dbl)  [unwired: 1 in]
            n174 = property class="DigNum (严格)"(reference=w334, "Val(Sgnl)"=w336) -> ()  [unwired: 1 in, 2 out]
            n175 = call "Add State to Queue.vi"("State(s) In (\"\")"=w338) -> ("States Out"=w339:string)  [unwired: 14 in]
          }
          event "清扫次数", "清扫间隔": Mouse Down {
            n176 = event-data() -> ("CtlRef"=w344:refnum<vi>)  [unwired: 1 in, 7 out]
            n177 = property class="DigNum (严格)"(reference=w344) -> (reference out=w341:refnum<vi>, "Value"=w342:u16)  [unwired: 1 in, 1 out]
            n178 = call "数字键盘.vi"("OldNumber"=w342) -> ("NewNumber"=w343:dbl)  [unwired: 1 in]
            n179 = property class="DigNum (严格)"(reference=w341, "Val(Sgnl)"=w343) -> ()  [unwired: 1 in, 2 out]
            n180 = call "Add State to Queue.vi"("State(s) In (\"\")"=w345) -> ("States Out"=w346:string)  [unwired: 14 in]
          }
          event "标液1": Value Change {
            n181 = event-data() -> ("NewVal"=w352:sgl)  [unwired: 1 in, 5 out]
            n182 = global read "多参数全局变量.vi" "MB session in"() -> (w353:refnum<class "MB_Master.lvclass">)
            n183 = call "纳清浊度_第一点校准数据写入.vi"("数值"=w352, "MB session in"=w353) -> ("error out"=w350:errorcluster)  [unwired: 8 in, 1 out]
            n184 = Enqueue Element At Opposite End(queue=w349, element=T1."Turb" ("元素"), error in (no error)=w350) -> ()  [unwired: 1 in, 3 out]
            n185 = call "Add State to Queue.vi"("State(s) In (\"\")"=w351) -> ("States Out"=w355:string)  [unwired: 14 in]
          }
          event "清扫模式": Value Change {
            n186 = event-data() -> ("NewVal"=w360:u16)  [unwired: 1 in, 5 out]
            n187 = global read "多参数全局变量.vi" "MB session in"() -> (w361:refnum<class "MB_Master.lvclass">)
            n188 = call "纳清浊度_清扫模式写入.vi"("清扫模式"=w360, "MB session in"=w361) -> ("error out"=w358:errorcluster)  [unwired: 8 in, 1 out]
            n189 = Enqueue Element At Opposite End(queue=w357, element=T1."Turb" ("元素"), error in (no error)=w358) -> ()  [unwired: 1 in, 3 out]
            n190 = call "Add State to Queue.vi"("State(s) In (\"\")"=w359) -> ("States Out"=w363:string)  [unwired: 14 in]
          }
          event "清扫次数": Value Change {
            n191 = event-data() -> ("NewVal"=w368:u16)  [unwired: 1 in, 5 out]
            n192 = global read "多参数全局变量.vi" "MB session in"() -> (w369:refnum<class "MB_Master.lvclass">)
            n193 = call "纳清浊度_清扫次数写入.vi"("数值"=w368, "MB session in"=w369) -> ("error out"=w366:errorcluster)  [unwired: 8 in, 1 out]
            n194 = Enqueue Element At Opposite End(queue=w365, element=T1."Turb" ("元素"), error in (no error)=w366) -> ()  [unwired: 1 in, 3 out]
            n195 = call "Add State to Queue.vi"("State(s) In (\"\")"=w367) -> ("States Out"=w371:string)  [unwired: 14 in]
          }
          event "清扫间隔": Value Change {
            n196 = event-data() -> ("NewVal"=w376:u16)  [unwired: 1 in, 5 out]
            n197 = global read "多参数全局变量.vi" "MB session in"() -> (w377:refnum<class "MB_Master.lvclass">)
            n198 = call "纳清浊度_清扫间隔写入.vi"("数值"=w376, "MB session in"=w377) -> ("error out"=w374:errorcluster)  [unwired: 8 in, 1 out]
            n199 = Enqueue Element At Opposite End(queue=w373, element=T1."Turb" ("元素"), error in (no error)=w374) -> ()  [unwired: 1 in, 3 out]
            n200 = call "Add State to Queue.vi"("State(s) In (\"\")"=w375) -> ("States Out"=w379:string)  [unwired: 14 in]
          }
          event "标液2": Value Change {
            n201 = event-data() -> ("NewVal"=w384:sgl)  [unwired: 1 in, 5 out]
            n202 = global read "多参数全局变量.vi" "MB session in"() -> (w385:refnum<class "MB_Master.lvclass">)
            n203 = call "纳清浊度_第二点校准数据写入.vi"("数值"=w384, "MB session in"=w385) -> ("error out"=w382:errorcluster)  [unwired: 8 in, 1 out]
            n204 = Enqueue Element At Opposite End(queue=w381, element=T1."Turb" ("元素"), error in (no error)=w382) -> ()  [unwired: 1 in, 3 out]
            n205 = call "Add State to Queue.vi"("State(s) In (\"\")"=w383) -> ("States Out"=w387:string)  [unwired: 14 in]
          }
          event "标液3": Value Change {
            n206 = event-data() -> ("NewVal"=w392:sgl)  [unwired: 1 in, 5 out]
            n207 = global read "多参数全局变量.vi" "MB session in"() -> (w393:refnum<class "MB_Master.lvclass">)
            n208 = call "纳清浊度_第三点校准数据写入.vi"("数值"=w392, "MB session in"=w393) -> ("error out"=w390:errorcluster)  [unwired: 8 in, 1 out]
            n209 = Enqueue Element At Opposite End(queue=w389, element=T1."Turb" ("元素"), error in (no error)=w390) -> ()  [unwired: 1 in, 3 out]
            n210 = call "Add State to Queue.vi"("State(s) In (\"\")"=w391) -> ("States Out"=w395:string)  [unwired: 14 in]
          }
          event "滤波设定": Value Change {
            n211 = event-data() -> ()  [unwired: 1 in, 6 out]
            n212 = flat-sequence {
              frame #0 {
                n213 = global read "断电保存变量.vi" "滤波设置"() -> (w401:T4)
                n214 = local read "滤波设定"() -> (w399:sgl)
                n215 = Bundle By Name(cluster=w401, "Turb"=w399) -> (w400:T4)
                n216 = global write "断电保存变量.vi" "滤波设置"(w400) -> ()
              }
              frame #1 {
                n217 = call "配置文件保存.vi"() -> ()  [unwired: 12 in]
              }
            }
            n218 = call "Add State to Queue.vi"("State(s) In (\"\")"=w396) -> ("States Out"=w398:string)  [unwired: 14 in]
          }
          event "量程": Value Change {
            n219 = event-data() -> ("NewVal"=w406:u16)  [unwired: 1 in, 5 out]
            n220 = global read "多参数全局变量.vi" "MB session in"() -> (w407:refnum<class "MB_Master.lvclass">)
            n221 = call "纳清浊度_量程写入.vi"("数值"=w406, "MB session in"=w407) -> ("error out"=w404:errorcluster)  [unwired: 8 in, 1 out]
            n222 = Enqueue Element At Opposite End(queue=w403, element=T1."Turb" ("元素"), error in (no error)=w404) -> ()  [unwired: 1 in, 3 out]
            n223 = call "Add State to Queue.vi"("State(s) In (\"\")"=w405) -> ("States Out"=w409:string)  [unwired: 14 in]
          }
          event "校准启动": Value Change {
            n224 = event-data() -> ()  [unwired: 1 in, 6 out]
            n225 = global read "纳清过程全局变量.vi" "浊度测试值"() -> (w412:T3)
            n226 = Unbundle By Name(w412) -> ("量程"=w411:u16)
            n227 = global read "多参数全局变量.vi" "MB session in"() -> (w413:refnum<class "MB_Master.lvclass">)
            n228 = call "纳清浊度_校准量程写入.vi"("数值"=w411, "MB session in"=w413) -> ("error out"=w410:errorcluster)  [unwired: 8 in, 1 out]
            n229 = global read "多参数全局变量.vi" "校准运行状态"() -> (w415:T7)
            n230 = Bundle By Name(cluster=w415, "Turb"=TRUE ("Cond")) -> (w416:T7)
            n231 = global write "多参数全局变量.vi" "校准运行状态"(w416) -> ()
            n232 = call "Add State to Queue.vi"("State(s) In (\"\")"=w420, "State(s) At Back (\"\")"="init: all\nCal: Place standard solution\n Cal: Calibration process\nidle" ("State(s) In (\"\")")) -> ("States Out"=w419:string)  [unwired: 13 in]
          }
          event "校准停止": Value Change {
            n233 = event-data() -> ()  [unwired: 1 in, 6 out]
            n234 = call "Add State to Queue.vi"("State(s) In (\"\")"="init: all\nCal: Over\nidle" ("State(s) In (\"\")")) -> ("States Out"=w422:string)  [unwired: 14 in]
          }
        }
      }
    }
  }
